vi "request error clear.vi"(8 "error in":errorcluster, 11 "async exec ref in":T1) -> (0 "error out":errorcluster, 3 "async exec ref out":T1)   [LabVIEW 2013]
uses:
  Runtime/async command notification.ctl
  async executor.lvlib
  <vilib>/NI/Tag Bus/table/data table.ctl
  <vilib>/NI/Tag Bus/table/data table.lvlib
  <vilib>/NI/Tag Bus/buffer exchange/buffer reference.ctl
  <vilib>/NI/Tag Bus/buffer exchange/tag bus buffer exchange.lvlib
  <vilib>/NI/Tag Bus Module Framework/runtime/error classification.ctl
  <vilib>/NI/Tag Bus Module Framework/runtime/TBM module execution interface.lvclass
  Runtime/async error info.ctl
  asynchronous executor reference.ctl
  message to executor.ctl
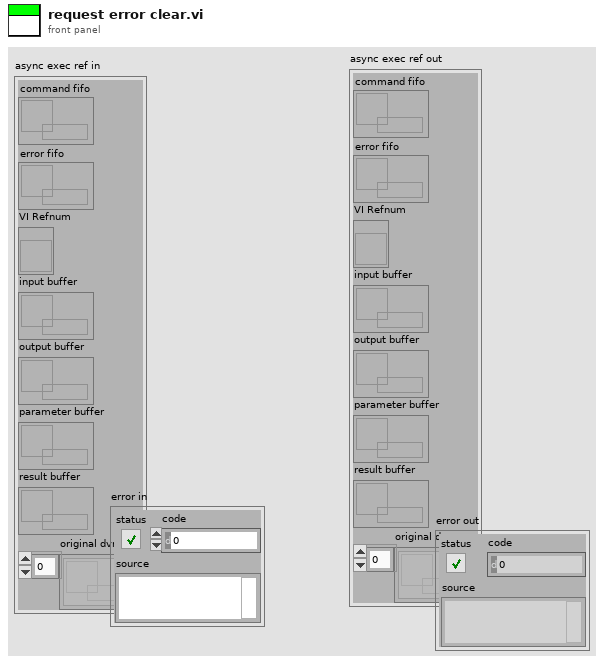
[diagram p1: front panel]
types:
  T1 = typedef "async executor.lvlib/asynchronous executor reference.ctl" = cluster{"command fifo":refnum<k33>, "error fifo":refnum<k33>, "VI Refnum":refnum<vi>, "input buffer":refnum<k33>, "output buffer":refnum<k33>, "parameter buffer":refnum<k33>, "result buffer":refnum<k33>, "original dvrs":T2[]}
  T2 = typedef "tag bus buffer exchange.lvlib/buffer reference.ctl" = refnum<data-value>
  T3 = typedef "async executor.lvlib/async command notification.ctl" = enum16{"stop", "input", "process", "output"}
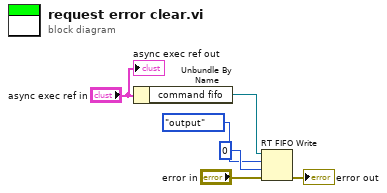
[diagram p0: block diagram]
diagram:
  n1 = Unbundle By Name("async exec ref in") -> ("command fifo"=w3:refnum<k33>)
  n2 = RT FIFO Write(0:w3, 1:async_command_notification."output" ("element"), 2:0 ("timeout in ms (0)"), 3:"error in") -> (11:→"error out":errorcluster)  [unwired: 1 in, 3 out]
  "async exec ref out" <- "async exec ref in"
